vi "Initialize.vi"(5 "instance":u8) -> (4 "subsystem":refnum<class "Single Address Space Collection.lvclass">, 6 "AddressSpace":refnum<class "AddressSpace.lvclass">)   [LabVIEW 2017, in "ScaleAndLimit.lvlib" / "AddressSpace.lvclass"]
doc: "Initializes the address space needed to comunicate through the Instruction Framework."
uses:
  AddressSpace.lvclass
  <instrlib>/_niInstr/Instruction Framework/v1/FPGA/Helper Classes/Single Address Space Collection/Single Address Space Collection.lvclass
  C:/Program Files (x86)/National Instruments/LabVIEW 2017/instr.lib/_niInstr/Instruction Framework/v1/FPGA/Interfaces/Address Space/Address Space.lvclass
  AddressSpace.lvclass/AddressSpace.ctl
  <vilib>/rvi/eio/common/nirviEmuReportErrorAndStop.vi
  <vilib>/rvi/DataTransferAndStorage/Container/Common/niFpgaContainerSetEmuInfo.vi
  <vilib>/rvi/DataTransferAndStorage/Container/Common/niFpgaContainerGetUniqueNameForEmu.vi
  <vilib>/rvi/LocalResourceManager/LocalResourceManager.xnode
  ScaleAndLimit.lvlib
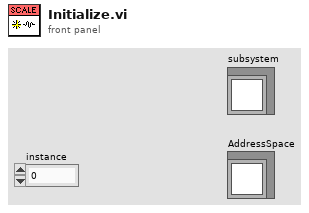
[diagram p1: front panel]
types:
  T1 = typedef "ScaleAndLimit.lvlib/LimitsRegisters.ctl" = cluster{"HighLimits":refnum<k21>, "LowLimits":refnum<k21>, "ClearLimits":refnum<k21>, "LimitsFlag":refnum<k21>}
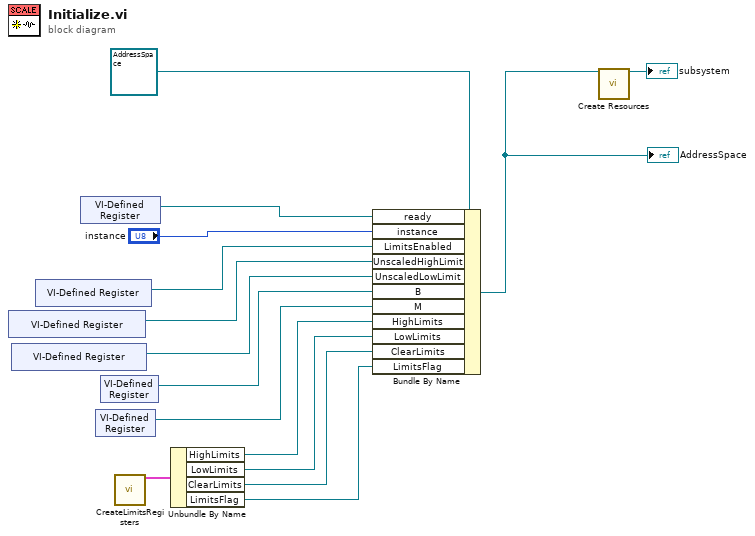
[diagram p0: block diagram]
diagram:
  n1 = xnode "VI-Defined Register"() -> ("Register Out"=w9:refnum<k21>)
  n2 = xnode "VI-Defined Register"() -> ("Register Out"=w8:refnum<k21>)
  n3 = xnode "VI-Defined Register"() -> ("Register Out"=w10:refnum<k21>)
  n4 = xnode "VI-Defined Register"() -> ("Register Out"=w11:refnum<k21>)
  n5 = xnode "VI-Defined Register"() -> ("Register Out"=w6:refnum<k21>)
  n6 = xnode "VI-Defined Register"() -> ("Register Out"=w7:refnum<k21>)
  n7 = call "CreateLimitsRegisters.vi"() -> ("LimitsRegisters"=w5:T1)  [unwired: 15 in]
  n8 = Unbundle By Name(w5) -> ("HighLimits"=w4:refnum<k21>, "LowLimits"=w3:refnum<k21>, "ClearLimits"=w2:refnum<k21>, "LimitsFlag"=w1:refnum<k21>)
  n9 = Bundle By Name(cluster=refnum<class "AddressSpace.lvclass"> refnum ("ScaleAndLimit.lvlib:AddressSpace.lvclass"), "ready"=w11, "instance"="instance", "LimitsEnabled"=w10, "UnscaledHighLimit"=w9, "UnscaledLowLimit"=w8, "B"=w7, "M"=w6, "HighLimits"=w4, "LowLimits"=w3, "ClearLimits"=w2, "LimitsFlag"=w1) -> (w12:refnum<class "AddressSpace.lvclass">)
  "AddressSpace" <- w12
  n10 = call <instrlib>:"Create Resources.vi"("address space"=w12) -> ("single address space collection"=→"subsystem":refnum<class "Single Address Space Collection.lvclass">)  [unwired: 14 in]
